vi "AFM_PI_control.vi"() -> ()   [LabVIEW 2017]
uses:
  controls/controlParams_tracktraj.ctl
  fpga_fp_interface_lib/fpga_interface_types/boolean_indicators.ctl
  <vilib>/rvi/Emulation/niFpgaGetClockAttributes.vi
  <vilib>/rvi/Emulation/niFpgaSctlEmulationGetInTimedLoop.vi
  <vilib>/rvi/Emulation/niFpgaEmulationReportErrorSimple.vi
  <vilib>/rvi/eio/common/nirviEmuTemplateMethod_errors.vi
  <vilib>/rvi/Emulation/niFpgaCriticalErrorInLSC.vi
  <vilib>/rvi/DataTransferAndStorage/Container/Common/niFpgaContainerExecOnDevCompGetState.vi
  <vilib>/rvi/Emulation/niFpgaEmulationIsFPGAContextNoSignature.vi
  <vilib>/rvi/DataTransferAndStorage/Container/Common/niFpgaContainerGetUniqueNameForEmu.vi
  <vilib>/rvi/Memory/Memory_Emulation/niFpgaMemoryEmulationCacheClearOnFirstRun.vi
  <vilib>/rvi/Memory/Memory_Emulation/nirvimemoryEmulationManagerCache_MakeExclusive.vi
  <vilib>/rvi/Memory/Memory_Emulation/niFpgaMemoryEmulationValidateCache.vi
  <vilib>/rvi/Memory/Memory_Emulation/nirvimemoryEmulationManagerCache_InsertValue.vi
  <vilib>/Utility/error.llb/Clear Errors.vi
  <vilib>/rvi/Memory/Memory_Emulation/nirvimemoryEmulationManagerCache_ReleaseExclusive.vi
  <vilib>/rvi/Memory/Memory_Emulation/nirvimemoryEmulationManagerCache_GetValue.vi
  <vilib>/rvi/Memory/Memory_Emulation/nirvimemoryEmulationManagerCache_SetValue.vi
  <vilib>/rvi/Emulation/niFpgaProcessEmulError.vi
  <vilib>/rvi/interface/RandomDataEmulation/niFpgaRandomDataHandleErrors.vi
  <vilib>/eio/EIONode/EIONode.xnode
  <vilib>/rvi/DataTransferAndStorage/Container/XNode/niFpgaContainer.xnode
  <vilib>/rvi/DataTransferAndStorage/Register/Emulation/niFpgaRegisterEmulationRefIn.vi
  <vilib>/rvi/interface/RandomDataEmulation/nirviRandomDataFpgaReadWriteTemplate.vi
  <vilib>/rvi/FXPMathLib/FxpSub/XNode/nifxpmath_Sub.xnode
  <vilib>/rvi/FXPMathLib/sim/FxpSim.dll
panel:
  out "boolean  indicators":T1
  in  "iters":i16=1
  out "rk":sgl
  in  "ControlParms":T2={"umax"=3.0, "y_ref(k)"=0.0, "Ki"=0.0, "y(k) (from plant)"=0.0, "ND"=0, "NS"=0, "u_Kx_ref(k)"=0.0, "du_max"=3.0, "NS_obs"=0, "NS_control"=0, "Kp"=0.0} {"Kp" format="%#_13g"; "du_max" format="%#_13g"; "u_Kx_ref(k)" format="%#_13g"; "Ki" format="%#_13g"; "y_ref(k)" format="%#_13g"; "umax" format="%#_13g"}
  in  "Settle Ticks":i16=1000
  in  "ymax":sgl=4.0 format="%#_13g"
  in  "TsTicks":i16
  out "Loop Ticks (benchmark)":i16
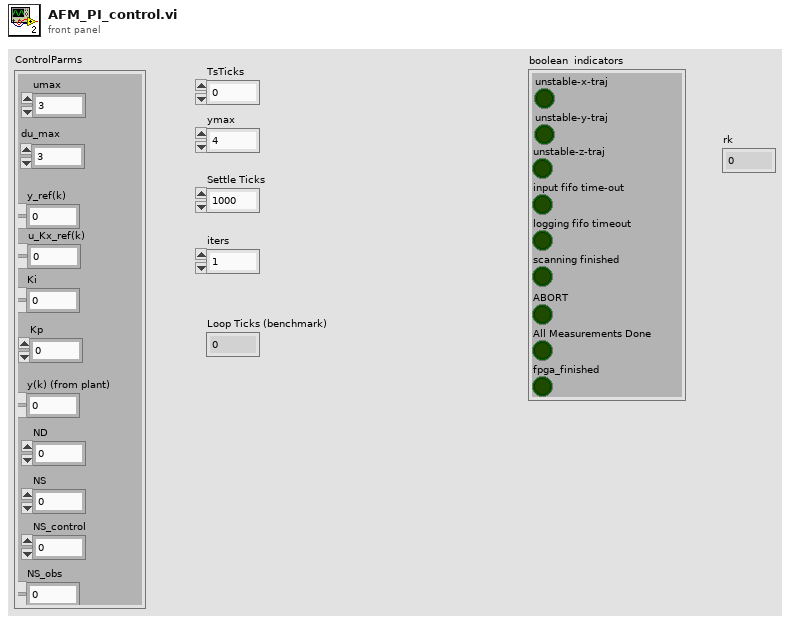
[diagram p1: front panel]
types:
  T1 = typedef "boolean_indicators.ctl" = cluster{"unstable-z-traj":bool, "input fifo time-out":bool, "logging fifo timeout":bool, "scanning finished":bool, "unstable-x-traj":bool, "unstable-y-traj":bool, "ABORT":bool, "All Measurements Done":bool, "fpga_finished":bool}
  T2 = typedef "controlParams_tracktraj.ctl" = cluster{"umax":sgl, "y_ref(k)":sgl, "Ki":sgl, "y(k) (from plant)":sgl, "ND":i16, "NS":i16, "u_Kx_ref(k)":sgl, "du_max":sgl, "NS_obs":i16, "NS_control":i16, "Kp":sgl}
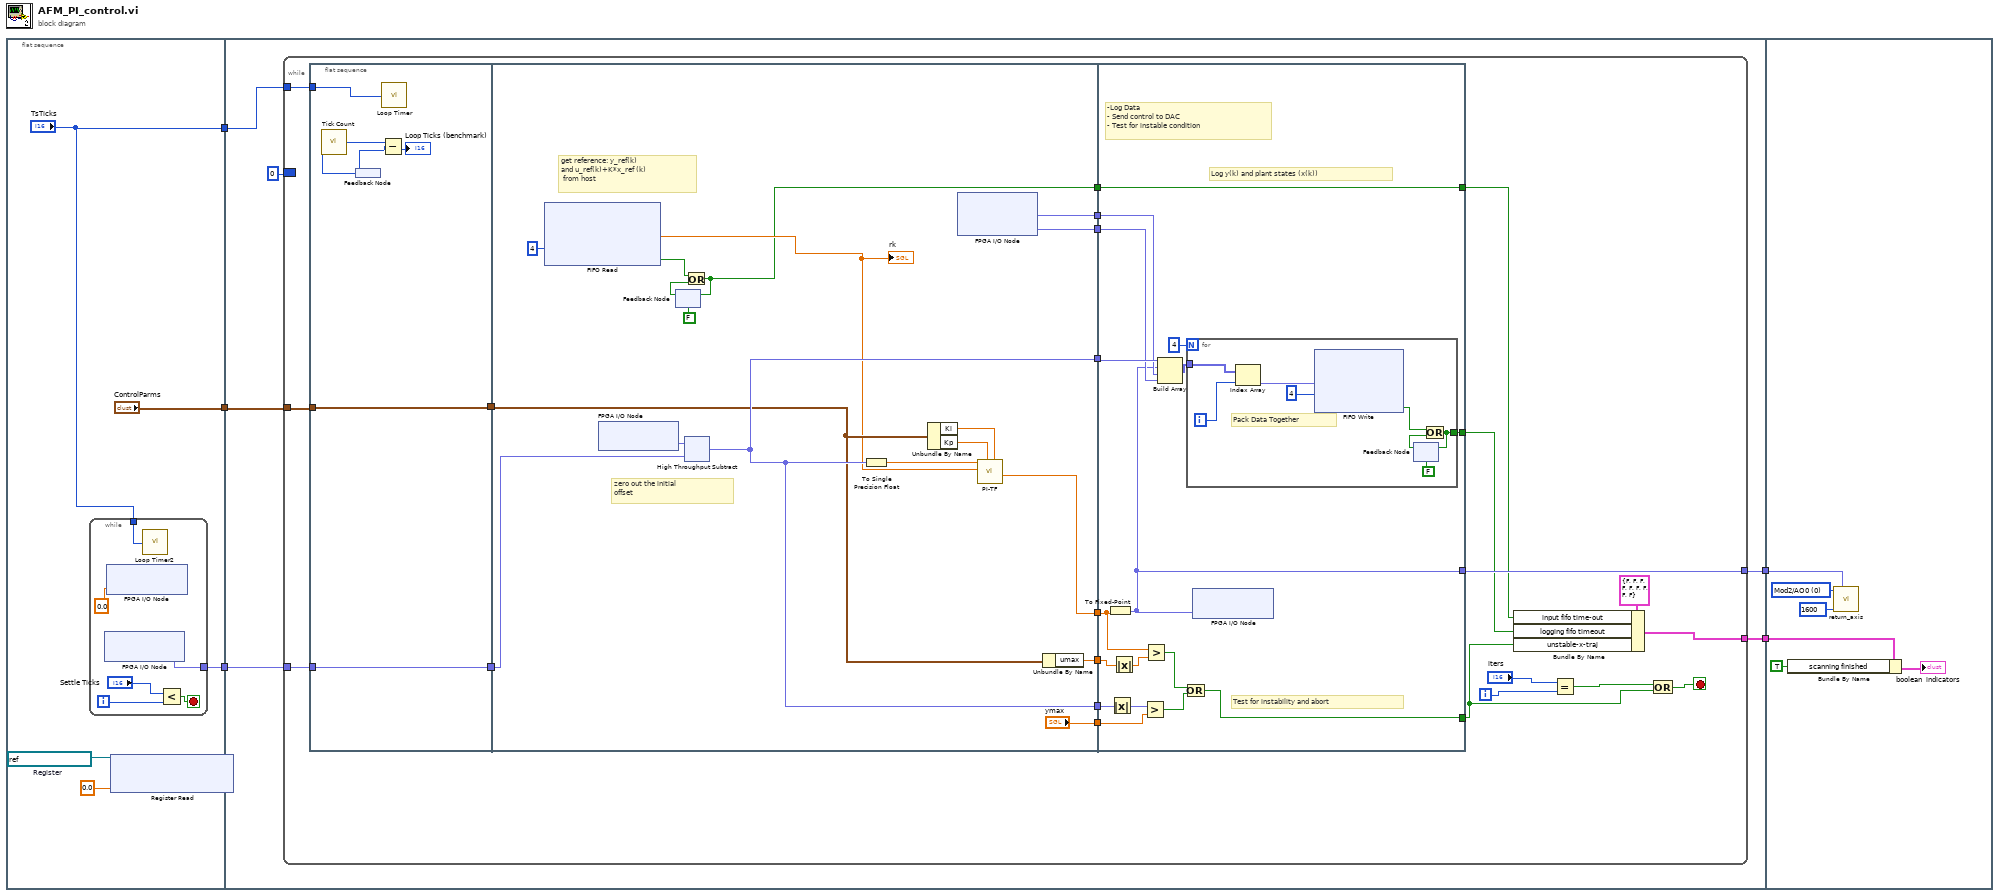
[diagram p0: block diagram]
diagram:
  n1 = flat-sequence {
    tunnel: ["TsTicks"] -> w5
    tunnel: [w10] -> w4
    tunnel: ["ControlParms"] -> w3
    tunnel: w5 -> [w21]
    tunnel: w4 -> [w20]
    tunnel: w3 -> [w19]
    tunnel: [w18] -> w2
    tunnel: [w17] -> w1
    tunnel: w2 -> [w98]
    tunnel: w1 -> [w95]
    frame #0 {
      w8 = refnum<k21> "accumulator"  # Register
      # "Load Matrix Data"
      n2 = while {
        tunnel: [w16] -> w10
        tunnel: "TsTicks" -> [w15]
        i -> [w11]
        stop <- w13 stop-if-true
        n3 = xnode "FPGA I/O Node"() -> ("Mod2/AI0"=w16:fxp<+/-,24,5>)  [unwired: 1 in, 1 out]
        n4 = xnode "FPGA I/O Node"("Mod1/AO0"=sgl 0.0) -> ()  [unwired: 1 in, 1 out]
        n5 = call "Loop Timer2"("Count(Ticks)"=w15) -> ()  [unwired: 1 out]
        n6 = Less?(x="Settle Ticks", y=w11) -> (x < y?=w13:bool)
      }
      n7 = xnode ("Register Read")("Data"=sgl 0.0, "Register In"=w8) -> ()  [unwired: 1 out]
    }
    frame #1 {
      n8 = while {
        border: i16 0 -> [_]
        tunnel: w21 -> [w44]
        tunnel: w20 -> [w42]
        tunnel: w19 -> [w39]
        tunnel: [w33] -> w18
        tunnel: [w27] -> w17
        i -> [w29]
        stop <- w30 stop-if-true
        n9 = flat-sequence {
          tunnel: w44 -> [w48]
          tunnel: w42 -> [w47]
          tunnel: [w47] -> w41
          tunnel: [w46] -> w40
          tunnel: w39 -> [w46]
          tunnel: [w58] -> w45
          tunnel: [w67] -> w43
          tunnel: w41 -> [w69]
          tunnel: w40 -> [w64]
          tunnel: [w67] -> w38
          tunnel: [w66] -> w37
          tunnel: ["ymax"] -> w36
          tunnel: [w63] -> w35
          tunnel: [w59] -> w34
          tunnel: [w52] -> w24
          tunnel: w45 -> [w82]
          tunnel: w43 -> [w84]
          tunnel: [w76] -> w28
          tunnel: w38 -> [w83]
          tunnel: w37 -> [w81]
          tunnel: w36 -> [w79]
          tunnel: w35 -> [w74]
          tunnel: w34 -> [w73]
          tunnel: [w72] -> w33
          tunnel: [w71] -> w25
          tunnel: [w70] -> w23
          tunnel: w24 -> [w70]
          frame #0 {
            n10 = call "Tick Count"() -> ("Tick Count(Ticks)"=w49:u32)
            n11 = feedback #1() -> (w50:u32)
            n12 = feedback-in #1(w49) -> ()
            n13 = Subtract(x=w49, y=w50) -> (x-y=→"Loop Ticks (benchmark)":u32)
            n14 = call "Loop Timer"("Count(Ticks)"=w48) -> ()  [unwired: 1 out]
          }
          frame #1 {
            # "get reference: y_ref(k)\nand u_ref(k)+K*x_ref (k)\n from host"
            # "zero out the initial \noffset"
            n15 = xnode ("FIFO Read")("Timeout"=i16 4) -> ("Element"=w56:sgl, "Timed Out?"=w53:bool)  [unwired: 1 in, 1 out]
            "rk" <- w56
            n16 = xnode "FPGA I/O Node"() -> ("Mod2/AI0"=w68:fxp<+/-,24,5>)  [unwired: 1 in, 1 out]
            n17 = feedback #2(FALSE) -> (w55:bool)
            n18 = Or(x=w53, y=w55) -> (x .or. y?=w52:bool)
            n19 = feedback-in #2(w52) -> ()
            n20 = xnode "High Throughput Subtract"("x"=w68, "y"=w69) -> ("x-y"=w67:fxp<+/-,40,6>)
            n21 = To Single Precision Float(number=w67) -> (single precision float=w62:sgl)
            n22 = Unbundle By Name(w64) -> ("Ki"=w61:sgl, "Kp"=w60:sgl)
            n23 = xnode "FPGA I/O Node"() -> ("Mod2/AI1"=w63:fxp<+/-,24,5>, "Mod2/AI2"=w59:fxp<+/-,24,5>)  [unwired: 2 in, 2 out]
            n24 = call "PI-TF.vi"("Ki"=w61, "Kp"=w60, "setpoint"=w56, "y(k)"=w62) -> ("u(k)"=w58:sgl)  [unwired: 7 in]
            n25 = Unbundle By Name(w64) -> ("umax"=w66:sgl)
          }
          frame #2 {
            # "Log y(k) and plant states (x(k))"
            # "-Log Data\n- Send control to DAC\n- Test for instable condition"
            # "Test for instability and abort"
            n26 = To Fixed-Point(number=w82) -> (fixed-point=w72:fxp<+/-,32,6>)  [unwired: 1 in]
            n27 = Absolute Value(x=w83) -> (abs(x)=w86:fxp<+,40,6>)
            n28 = Absolute Value(x=w81) -> (abs(x)=w80:sgl)
            n29 = Greater?(x=w86, y=w79) -> (0:w77:bool)
            n30 = Greater?(x=w82, y=w80) -> (0:w78:bool)
            n31 = Build Array(w84, w72, w74, w73) -> (w85:fxp<+/-,40,6>[])
            n32 = Or(x=w78, y=w77) -> (x .or. y?=w76:bool)
            n33 = for {
              N: 4 -> [_]
              tunnel: w85 -> [w92]
              tunnel: [w87] -> w71
              i -> [w93]
              # "Pack Data Together"
              n34 = Index Array(array=w92, index=w93) -> (element=w91:fxp<+/-,40,6>)
              n35 = xnode ("FIFO Write")("Element"=w91, "Timeout"=i16 4) -> ("Timed Out?"=w90:bool)  [unwired: 1 in, 1 out]
              n36 = feedback #3(FALSE) -> (w89:bool)
              n37 = Or(x=w90, y=w89) -> (x .or. y?=w87:bool)
              n38 = feedback-in #3(w87) -> ()
            }
            n39 = xnode "FPGA I/O Node"("Mod1/AO0"=w72) -> ()  [unwired: 1 in, 1 out]
          }
        }
        n40 = Bundle By Name(cluster=T1 {"unstable-z-traj"=FALSE, "input fifo time-out"=FALSE, "logging fifo timeout"=FALSE, "scanning finished"=FALSE, "unstable-x-traj"=FALSE, "unstable-y-traj"=FALSE, "ABORT"=FALSE, "All Measurements Done"=FALSE, "fpga_finished"=FALSE} ("boolean  indicators"), "input fifo time-out"=w23, "logging fifo timeout"=w25, "unstable-x-traj"=w28) -> (w27:T1)
        n41 = Equal?(x="iters", y=w29) -> (x = y?=w31:bool)
        n42 = Compound Arithmetic op=OR(w31, w28) -> (w30:bool)
      }
    }
    frame #2 {
      w99 = i16 0 items=["Mod2/AO0", "Mod2/AO1", "Mod2/AO2", "Mod2/AO3", ""] ("DAC-select")
      n43 = Bundle By Name(cluster=w95, "scanning finished"=TRUE) -> (→"boolean  indicators":T1)
      n44 = call "return_axis.vi"("u(0)"=w98, "TsTicks"=u32 1600, "DAC-select"=w99) -> ()  [unwired: 9 in]
    }
  }
